vi "Initialize_Devices_Main_v1.vi"(8 "error in":errorcluster, 11 "Resource Address":T4={"ZI Address"="DEV714", "VISA Keithley"="", "VISA Arduino PG"=""}) -> (0 "error out":errorcluster, 3 "Resources":T1 {"ZI ModHandle"."ModHandle" format="0x%08x"; "ZI ModHandle"."Conn" format="0x%08x"; "ZI Handle"."Handle" format="0x%08x"; "ZI Handle"."Conn" format="0x%08x"})   [LabVIEW 2021]
uses:
  Resources.ctl
  <instrlib>/Zurich Instruments LabOne/Public/ziTypeHandle.ctl
  <instrlib>/Zurich Instruments LabOne/Public/Modules/ziTypeModHandle.ctl
  <instrlib>/Zurich Instruments LabOne/Public/Modules/ziTypeModEnum.ctl
  <instrlib>/Keithley 622x LV 2009/Utility/Typedefs/KE622x -- Instrument Type.ctl
  <instrlib>/Keithley 622x LV 2009/Utility/Typedefs/KE622x -- Serial Port Settings.ctl
  <instrlib>/Zurich Instruments LabOne/Zurich Instruments LabOne.lvlib
  <instrlib>/Keithley 622x LV 2009/Keithley 622x.lvlib
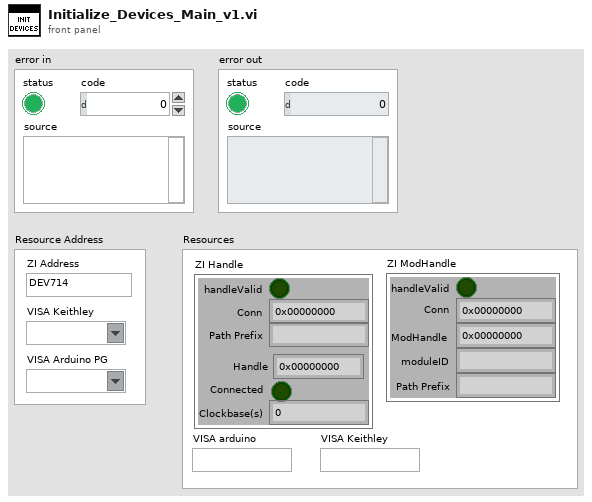
[diagram p1: front panel]
types:
  T1 = typedef "Resources.ctl" = cluster{"ZI Handle":T2, "ZI ModHandle":T3, "VISA arduino":refnum<visa-resource-name>, "VISA Keithley":refnum<visa-resource-name>}
  T2 = typedef "Zurich Instruments LabOne.lvlib/ziTypeHandle.ctl" = cluster{"handleValid":bool, "Conn":u64, "Path Prefix":string, "Handle":u64, "Connected":bool, "Clockbase(s)":dbl}
  T3 = typedef "Zurich Instruments LabOne.lvlib/ziTypeModHandle.ctl" = cluster{"handleValid":bool, "Conn":u64, "ModHandle":u64, "moduleID":string, "Path Prefix":string}
  T4 = cluster{"ZI Address":string, "VISA Keithley":refnum<visa-resource-name>, "VISA Arduino PG":refnum<visa-resource-name>}
  T5 = typedef "Keithley 622x.lvlib/KE622x -- Serial Port Settings.ctl" = cluster{"Read Term Char":enum16{"CR", "LF", "CR + LF", "LF + CR"}, "Baud Rate":enum16{"300", "600", "1200", "2400", "4800", "9600", "19200", "38400", "57600", "115200"}, "Flow Control\n(XON / XOFF)":enum16{"Off", "On"}}
  T6 = typedef "Keithley 622x.lvlib/KE622x -- Instrument Type.ctl" = enum16{"KE6220", "KE6221"}
  T7 = typedef "Zurich Instruments LabOne.lvlib/ziTypeModEnum.ctl" = u16
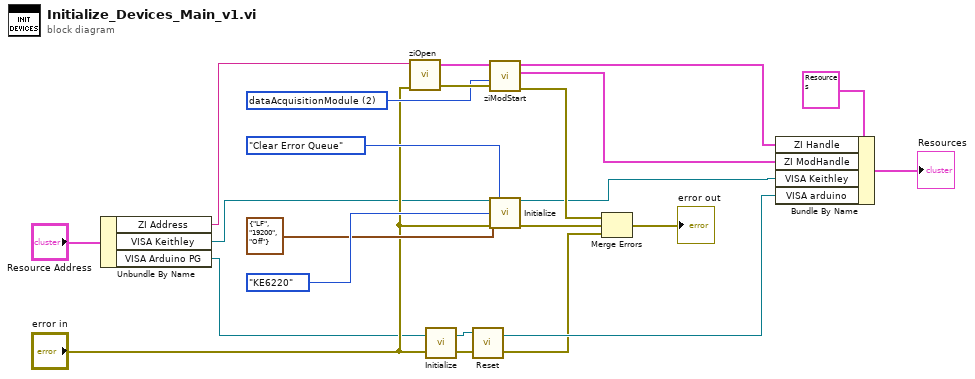
[diagram p0: block diagram]
diagram:
  w21 = T7 2 items=["sweep", "scopeModule", "dataAcquisitionModule", "pidAdvisor", "awgModule", "impedanceModule", "multiDeviceSyncModule", "zoomFFT", "trigger", "deviceSettings", "record", "precompensationAdvisor"] ("module Id")
  n1 = Unbundle By Name("Resource Address") -> ("ZI Address"=w10:string, "VISA Keithley"=w11:refnum<visa-resource-name>, "VISA Arduino PG"=w12:refnum<visa-resource-name>)
  n2 = call <instrlib>:"ziOpen.vi"("Error In"="error in", "Address"=w10) -> ("Error Out"=w22:errorcluster, "HandleOut"=w23:T2)  [unwired: 2 in, 1 out]
  n3 = call <instrlib>:"Initialize.vi"("error in"="error in", "VISA arduino in"=w12) -> ("error out"=w3:errorcluster, "VISA arduino out"=w4:refnum<visa-resource-name>)
  n4 = call "Reset.vi"("error in"=w3, "VISA arduino in"=w4) -> ("error out"=w1:errorcluster, "VISA arduino out"=w2:refnum<visa-resource-name>)  [unwired: 1 in]
  n5 = call <instrlib>:"ziModStart.vi"("Error In"=w22, "module Id"=w21, "Handle In"=w23) -> ("Error Out"=w17:errorcluster, "ModHandle Out"=w6:T3, "Handle Out"=w5:T2)  [unwired: 6 in]
  n6 = call <instrlib>:"Initialize.vi"("VISA resource name"=w11, "Error Queue Option"=enum16{"Clear Error Queue", "Error Query"}."Clear Error Queue", "RS-232 Settings"=T5 {"Read Term Char"=enum."LF", "Baud Rate"=enum."19200", "Flow Control\n(XON / XOFF)"=enum."Off"}, "Instrument Type"=KE622x_--_Instrument_Type."KE6220", "error in (no error)"="error in") -> ("VISA resource name out"=w7:refnum<visa-resource-name>, "error out"=w16:errorcluster)  [unwired: 9 in]
  n7 = Merge Errors(w17, w16, w1) -> (→"error out":errorcluster)
  n8 = Bundle By Name(cluster=T1 {"ZI Handle"={"handleValid"=FALSE, "Conn"=0, "Path Prefix"="", "Handle"=0, "Connected"=FALSE, "Clockbase(s)"=0.0}, "ZI ModHandle"={"handleValid"=FALSE, "Conn"=0, "ModHandle"=0, "moduleID"="", "Path Prefix"=""}, "VISA arduino"="", "VISA Keithley"=""} ("Resources"), "ZI Handle"=w5, "ZI ModHandle"=w6, "VISA Keithley"=w7, "VISA arduino"=w2) -> (→"Resources":T1)
